vi "ReportPart_A131258.vi"(8 "error in":errorcluster, 9 "索引":i32, 10 "合格":T1, 11 "report in":refnum<class "NI_report.lvclass">) -> (0 "error out 2":errorcluster caption="error out", 3 "report out":refnum<class "NI_report.lvclass">)   [LabVIEW 2020]
uses:
  <vilib>/Utility/NIReport.llb/NI_report.lvclass
  OK.ctl
  <vilib>/Utility/NIReport.llb/image depth.ctl
  <vilib>/addons/_office/_exclsub.llb/font.ctl
  Global_Variable/A131258.vi
  <vilib>/Utility/NIReport.llb/Append Report Text (str wrap).vi
  Global_Variable/Global.vi
  <vilib>/addons/_office/word.llb/Word Easy Table (str).vi
  <vilib>/Utility/NIReport.llb/NI_ReportGenerationCore.lvlib
  <vilib>/Utility/NIReport.llb/Word/NI_Word.lvclass
  <vilib>/addons/_office/NI_ReportGenerationToolkit.lvlib
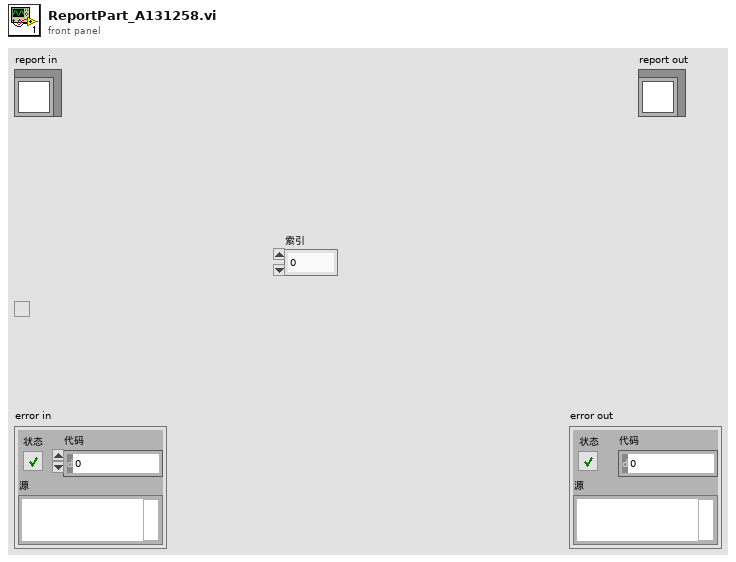
[diagram p1: front panel]
types:
  T1 = typedef "OK.ctl" = bool
  T2 = cluster{"Charset (-1)":i16, "Weight (-1)":i16, "Name":string, "Size":string}
  T3 = cluster{"Italic":enum16{"Italic Unchanged", "Italic On", "Italic Off"}, "Strike Through":enum16{"Strike Through Unchanged", "Strike Through On", "Strike Through Off"}, "Underline":enum16{"Underline Unchanged", "Underline On", "Underline Off"}, "Bold":enum16{"Bold Unchanged", "Bold On", "Bold Off"}}
  T4 = typedef "NI_ReportGenerationToolkit.lvlib/font.ctl" = cluster{"font name":string, "font size":dbl, "bold":u16, "italic":u16, "underline":u16, "strike through":u16, "font color":u32}
  T5 = typedef "NI_ReportGenerationCore.lvlib/image depth.ctl" = u16
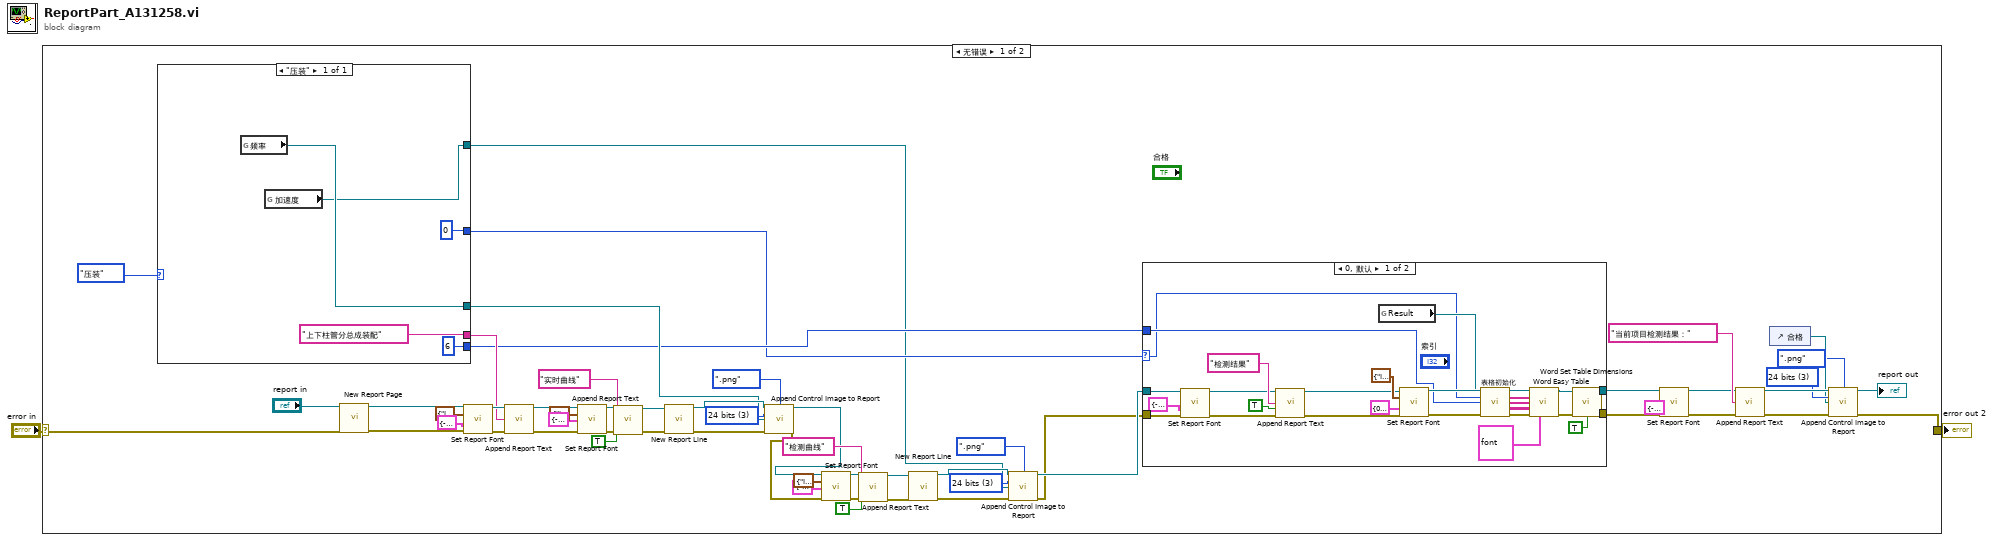
[diagram p0: block diagram]
diagram:
  n1 = case shown="无错误" "error in" {
    selector: "error in" -> [w40 w93]
    tunnel: [w34 w93] -> w1
    frame No Error {
      w17 = T5 3 items=["B&W", "4 bits", "8 bits", "24 bits"] ("image depth")
      w32 = T5 3 items=["B&W", "4 bits", "8 bits", "24 bits"] ("image depth")
      w57 = T5 3 items=["B&W", "4 bits", "8 bits", "24 bits"] ("image depth")
      n2 = case shown="\"压装\"" enum32{"压装"}."压装" ("试验项目") {
        tunnel: [w89] -> w23
        tunnel: ["上下柱管分总成装配" ("text")] -> w53
        tunnel: [6 ("长度")] -> w22
        tunnel: [0 ("长度")] -> w21
        tunnel: [w88] -> w3
        frame "压装" {
          n3 = global read "A131258.vi" "频率"() -> (w89:refnum<vi>)
          n4 = global read "A131258.vi" "加速度"() -> (w88:refnum<vi>)
        }
      }
      n5 = call-dynamic "New Report Page.vi"("report in"="report in", "error in (no error)"=w40) -> ("report out"=w38:refnum<class "NI_report.lvclass">, "error out"=w39:errorcluster)  [unwired: 12 in]
      n6 = call-dynamic "Set Report Font.vi"("report in"=w38, "text options"=T3 {"Italic"=enum."Italic Unchanged", "Strike Through"=enum."Strike Through Unchanged", "Underline"=enum."Underline Unchanged", "Bold"=enum."Bold On"}, "font settings"=T2 {"Charset (-1)"=-1, "Weight (-1)"=-1, "Name"="楷体", "Size"="16 "}, "error in (no error)"=w39) -> ("report out"=w56:refnum<class "NI_report.lvclass">, "error out"=w55:errorcluster)  [unwired: 9 in, 1 out]
      n7 = call-poly <vilib>:"Append Report Text.vi"("report in"=w56, "text"=w53, "error in (no error)"=w55) -> ("report out"=w51:refnum<class "NI_report.lvclass">, "error out"=w50:errorcluster)  [unwired: 9 in, 2 out]
      n8 = call-dynamic "Set Report Font.vi"("report in"=w51, "text options"=T3 {"Italic"=enum."Italic Unchanged", "Strike Through"=enum."Strike Through Unchanged", "Underline"=enum."Underline Unchanged", "Bold"=enum."Bold Off"}, "font settings"=T2 {"Charset (-1)"=-1, "Weight (-1)"=-1, "Name"="宋体", "Size"="12 "}, "error in (no error)"=w50) -> ("report out"=w47:refnum<class "NI_report.lvclass">, "error out"=w44:errorcluster)  [unwired: 9 in, 1 out]
      n9 = call-poly <vilib>:"Append Report Text.vi"("report in"=w47, "text"="实时曲线", "append on new line? (F)"=TRUE, "error in (no error)"=w44) -> ("report out"=w46:refnum<class "NI_report.lvclass">, "error out"=w45:errorcluster)  [unwired: 8 in, 2 out]
      n10 = call-dynamic "New Report Line.vi"("report in"=w46, "error in (no error)"=w45) -> ("report out"=w58:refnum<class "NI_report.lvclass">, "error out"=w59:errorcluster)  [unwired: 12 in]
      n11 = call-dynamic "Append Control Image to Report.vi"("report in"=w58, "image file type (.jpg)"=enum16{".jpg", ".png"}.".png", "image depth"=w57, "ctrl reference"=w23, "error in (no error)"=w59) -> ("report out"=w5:refnum<class "NI_report.lvclass">, "error out"=w4:errorcluster)  [unwired: 7 in, 2 out]
      n12 = call-dynamic "Set Report Font.vi"("report in"=w5, "text options"=T3 {"Italic"=enum."Italic Unchanged", "Strike Through"=enum."Strike Through Unchanged", "Underline"=enum."Underline Unchanged", "Bold"=enum."Bold Off"}, "font settings"=T2 {"Charset (-1)"=-1, "Weight (-1)"=-1, "Name"="宋体", "Size"="12 "}, "error in (no error)"=w4) -> ("report out"=w14:refnum<class "NI_report.lvclass">, "error out"=w11:errorcluster)  [unwired: 9 in, 1 out]
      n13 = call-poly <vilib>:"Append Report Text.vi"("report in"=w14, "text"="检测曲线", "append on new line? (F)"=TRUE, "error in (no error)"=w11) -> ("report out"=w13:refnum<class "NI_report.lvclass">, "error out"=w12:errorcluster)  [unwired: 8 in, 2 out]
      n14 = call-dynamic "New Report Line.vi"("report in"=w13, "error in (no error)"=w12) -> ("report out"=w18:refnum<class "NI_report.lvclass">, "error out"=w19:errorcluster)  [unwired: 12 in]
      n15 = call-dynamic "Append Control Image to Report.vi"("report in"=w18, "image file type (.jpg)"=enum16{".jpg", ".png"}.".png", "image depth"=w17, "ctrl reference"=w3, "error in (no error)"=w19) -> ("report out"=w7:refnum<class "NI_report.lvclass">, "error out"=w6:errorcluster)  [unwired: 7 in, 2 out]
      n16 = case shown="0, 默认" w21 {
        selector: w21 -> [w60 _]
        tunnel: w7 -> [w81 w87]
        tunnel: w6 -> [w79 w86]
        tunnel: [w66 w87] -> w25
        tunnel: [w65 w86] -> w24
        tunnel: w22 -> [w61 _]
        frame 0, Default {
          n17 = call-dynamic "Set Report Font.vi"("report in"=w81, "font settings"=T2 {"Charset (-1)"=-1, "Weight (-1)"=-1, "Name"="宋体", "Size"="12 "}, "error in (no error)"=w79) -> ("report out"=w82:refnum<class "NI_report.lvclass">, "error out"=w80:errorcluster)  [unwired: 10 in, 1 out]
          n18 = call-poly <vilib>:"Append Report Text.vi"("report in"=w82, "text"="检测结果", "append on new line? (F)"=TRUE, "error in (no error)"=w80) -> ("report out"=w64:refnum<class "NI_report.lvclass">, "error out"=w63:errorcluster)  [unwired: 8 in, 2 out]
          n19 = global read "Global.vi" "Result"() -> (w62:refnum<vi>)
          n20 = call-dynamic "Set Report Font.vi"("report in"=w64, "text options"=T3 {"Italic"=enum."Italic Unchanged", "Strike Through"=enum."Strike Through Unchanged", "Underline"=enum."Underline Unchanged", "Bold"=enum."Bold Unchanged"}, "font settings"=T2 {"Charset (-1)"=0, "Weight (-1)"=-1, "Name"="微软雅黑", "Size"="12 "}, "error in (no error)"=w63) -> ("report out"=w68:refnum<class "NI_report.lvclass">, "error out"=w67:errorcluster)  [unwired: 9 in, 1 out]
          n21 = call "表格初始化.vi"("表格引用"=w62, "索引"=w60, "长度"=w61, "错误输入（无错误）"=w67) -> ("行首字符串[]"=w70:string[], "列首字符串[]"=w69:string[], "文本数据"=w72:string[][], "错误输出"=w75:errorcluster)  [unwired: 7 in, 1 out]
          n22 = call-poly <vilib>:"Word Easy Table.vi"("report in"=w68, "row headers"=w70, "column headers"=w69, "data"=w72, "error in (no error)"=w75, "font"=T4 {"font name"="宋体", "font size"=12.0, "bold"=2, "italic"=2, "underline"=2, "strike through"=2, "font color"=16777216}) -> ("report out"=w73:refnum<class "NI_report.lvclass">, "error out"=w74:errorcluster)  [unwired: 7 in, 1 out]
          n23 = call <vilib>:"Word Set Table Dimensions.vi"("report in"=w73, "error in (no error)"=w74, "fit to page width? (F)"=TRUE) -> ("report out"=w66:refnum<class "NI_report.lvclass">, "error out"=w65:errorcluster)  [unwired: 11 in]
        }
        frame -1 {
        }
      }
      n24 = call-dynamic "Set Report Font.vi"("report in"=w25, "font settings"=T2 {"Charset (-1)"=-1, "Weight (-1)"=-1, "Name"="宋体", "Size"="16 "}, "error in (no error)"=w24) -> ("report out"=w29:refnum<class "NI_report.lvclass">, "error out"=w30:errorcluster)  [unwired: 10 in, 1 out]
      n25 = call-poly <vilib>:"Append Report Text.vi"("report in"=w29, "text"="当前项目检测结果：", "error in (no error)"=w30) -> ("report out"=w37:refnum<class "NI_report.lvclass">, "error out"=w35:errorcluster)  [unwired: 9 in, 2 out]
      n26 = control-ref of="合格"() -> (w31:refnum<vi>)
      n27 = call-dynamic "Append Control Image to Report.vi"("report in"=w37, "image file type (.jpg)"=enum16{".jpg", ".png"}.".png", "image depth"=w32, "ctrl reference"=w31, "error in (no error)"=w35) -> ("report out"=→"report out":refnum<class "NI_report.lvclass">, "error out"=w34:errorcluster)  [unwired: 7 in, 2 out]
    }
    frame Error {
    }
  }
  "error out 2" <- w1
